vi "Clear File Contents.vi"(8 "error in (no error)":errorcluster, 11 "Macro in":refnum<class "Macro.lvclass">) -> (0 "error out":errorcluster, 3 "Macro out":refnum<class "Macro.lvclass">)   [LabVIEW 2020, in "MacroAssert.lvlib" / "Macro.lvclass"]
uses:
  Macro.lvclass
  Macro.lvclass/Macro.ctl
  <vilib>/Utility/config.llb/NI_LVConfig.lvlib
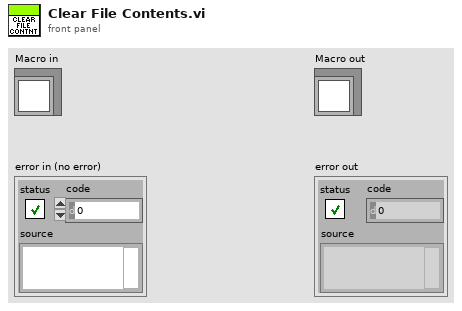
[diagram p1: front panel]
types:
  T1 = typedef "NI_LVConfig.lvlib/Config Data RefNum.ctl" = refnum<k1>
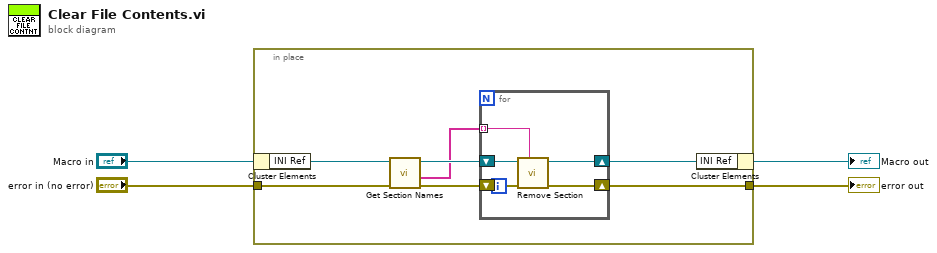
[diagram p0: block diagram]
diagram:
  n1 = in-place {
    in-place-border: "error in (no error)" -> [w8]
    in-place-border: [w5] -> w2
    n2 = in-place-cluster #1("Macro in") -> ("INI Ref"=w7:T1)
    n3 = call <vilib>:"Get Section Names.vi"("error in (no error)"=w8, "refnum"=w7) -> ("error out"=w11:errorcluster, "section names"=w9:string[], "refnum out"=w10:T1)  [unwired: 7 in]
    n4 = for {
      shift-right: [w12] -> w5
      shift-left: w11 -> [w15]
      shift-right: [w13] -> w6
      shift-left: w10 -> [w16]
      tunnel: w9 -> [w14] mode=indexing
      n5 = call <vilib>:"Remove Section.vi"("section"=w14, "error in (no error)"=w15, "refnum"=w16) -> ("error out"=w12:errorcluster, "refnum out"=w13:T1)  [unwired: 6 in, 1 out]
    }
    n6 = in-place-cluster #1("INI Ref"=w6) -> (→"Macro out":refnum<class "Macro.lvclass">)
  }
  "error out" <- w2
